vi "Periodic Tasks.vi"(8 "error in":errorcluster) -> ()   [LabVIEW 2019]
doc: "This VI runs in parallel to other tasks. It can contain as many user-defined periodic loops as you need. These can carry out PID or other sorts of timed response."
uses:
  <vilib>/Rock Robotics/WPI/ThirdParty/Phoenix-LabVIEW/Motor Controller/Get/CTRE_Phoenix_MotorController_GetSelectedSensorData.vi
  <vilib>/Rock Robotics/Network Tables/NT Write Number.vi
  <vilib>/Rock Robotics/WPI/ThirdParty/Phoenix-LabVIEW/Motor Controller/Get/CTRE_Phoenix_MotorController_GetQuadratureData.vi
  <vilib>/Rock Robotics/Network Tables/NT Read Number.vi
  <vilib>/Rock Robotics/Network Tables/NT Read Boolean.vi
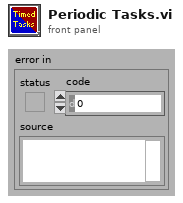
[diagram p1: front panel]
types:
  T1 = typedef "WPI_MotorControlDeviceRef.ctl" = cluster{"DeviceStatus":errorcluster, "Type":T2, "PWM":cluster{"PWM Channel":T3, "DeadBand":T4}, "CAN":cluster{"Device Number":u8, "SetOutput VI Ref":variant, "GetOutput VI Ref":variant, "Enable VI Ref":variant, "Disable VI Ref":variant, "Data":variant}, "Invert":bool, "DIO PWM":cluster{"PWM \"Enable\" Channel":T3, "DIOChannel":T5, "PWM Rate":dbl}}
  T2 = typedef "WPI_MotorControlType.ctl" = enum16{"PWM", "CAN", "DIO PWM"}
  T3 = typedef "FPGA_DIOPWMChannel.ctl" = enum8{"PWM 0", "PWM 1", "PWM 2", "PWM 3", "PWM 4", "PWM 5", "PWM 6", "PWM 7", "PWM 8", "PWM 9", "PWM MXP 0", "PWM MXP 1", "PWM MXP 2", "PWM MXP 3", "PWM MXP 4", "PWM MXP 5", "PWM MXP 6", "PWM MXP 7", "PWM MXP 8", "PWM MXP 9", "Invalid"}
  T4 = typedef "WPI_PWMDeadband.ctl" = cluster{"Name":string, "maxPositivePwm":i32, "minPositivePwm":i32, "centerPwm":i32, "maxNegativePwm":i32, "minNegativePwm":i32, "angularRange":u16}
  T5 = typedef "FPGA_DIOChannel.ctl" = enum8{"DIO 0", "DIO 1", "DIO 2", "DIO 3", "DIO 4", "DIO 5", "DIO 6", "DIO 7", "DIO 8", "DIO 9", "DIO MXP 0", "DIO MXP 1", "DIO MXP 2", "DIO MXP 3", "DIO MXP 4", "DIO MXP 5", "DIO MXP 6", "DIO MXP 7", "DIO MXP 8", "DIO MXP 9", "DIO MXP 10", "DIO MXP 11", "DIO MXP 12", "DIO MXP 13", "DIO MXP 14", "DIO MXP 15", "SPI Port CS1", "SPI Port CS2", "SPI Port CS3", "SPI Port MISO", "SPI Port MOSI", "Invalid"}
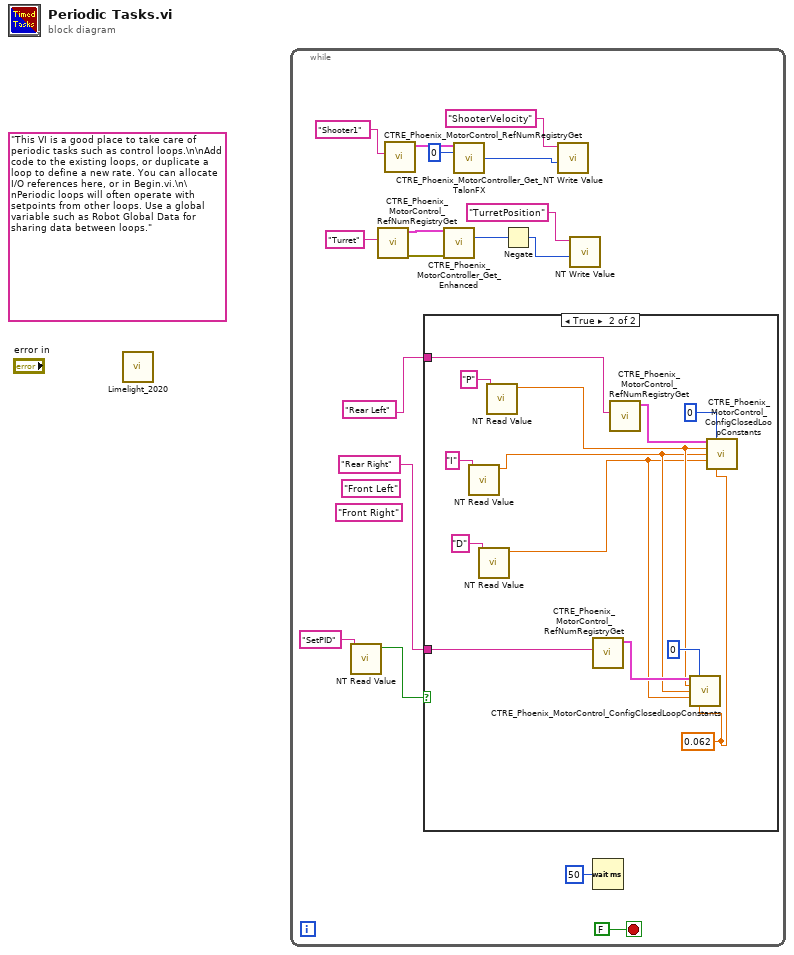
[diagram p0: block diagram]
diagram:
  (unwired) "This VI is a good place to take care of periodic tasks such as control loops.\n\nAdd code to the existing loops, or duplicate a loop to define a new rate. You can allocate I/O references here, or in Begin.vi.\n\nPeriodic loops will often operate with setpoints from other loops. Use a global variable such as Robot Global Data for sharing data between loops."
  n1 = call "Limelight_2020.vi"() -> ()  [unwired: 12 in]
  n2 = while {
    stop <- FALSE stop-if-true
    (unwired) "Front Right" ("refnum name")
    (unwired) "Front Left" ("refnum name")
    n3 = call-poly <vilib>:"NT Read Value.vi"("Name"="SetPID") -> ("Boolean"=w3:bool)  [unwired: 9 in, 1 out]
    n4 = call <vilib>:"CTRE_Phoenix_MotorControl_RefNumRegistryGet.vi"("refnum name"="Turret") -> ("error out"=w8:errorcluster, "PhoenixMotorControlDevRef"=w9:T1)  [unwired: 9 in]
    n5 = call <vilib>:"CTRE_Phoenix_MotorControl_RefNumRegistryGet.vi"("refnum name"="Shooter1") -> ("PhoenixMotorControlDevRef"=w15:T1)  [unwired: 9 in, 1 out]
    n6 = case shown="True" w3 {
      tunnel: "Rear Right" ("refnum name") -> [_ w25]
      tunnel: "Rear Left" ("refnum name") -> [_ w22]
      frame False {
      }
      frame True {
        w18 = 0.062 ("F")
        n7 = call-poly <vilib>:"NT Read Value.vi"("Name"="I") -> ("Numeric"=w20:dbl)  [unwired: 9 in, 1 out]
        n8 = call-poly <vilib>:"NT Read Value.vi"("Name"="D") -> ("Numeric"=w19:dbl)  [unwired: 9 in, 1 out]
        n9 = call-poly <vilib>:"NT Read Value.vi"("Name"="P") -> ("Numeric"=w21:dbl)  [unwired: 9 in, 1 out]
        n10 = call <vilib>:"CTRE_Phoenix_MotorControl_RefNumRegistryGet.vi"("refnum name"=w25) -> ("PhoenixMotorControlDevRef"=w24:T1)  [unwired: 9 in, 1 out]
        n11 = call <vilib>:"CTRE_Phoenix_MotorControl_RefNumRegistryGet.vi"("refnum name"=w22) -> ("PhoenixMotorControlDevRef"=w23:T1)  [unwired: 9 in, 1 out]
        n12 = call <vilib>:"CTRE_Phoenix_MotorControl_ConfigClosedLoopConstants.vi"("PhoenixMotorControlDevRef"=w24, "slotIdx"=0, "P"=w21, "I"=w20, "D"=w19, "F"=w18) -> ()  [unwired: 8 in, 2 out]
        n13 = call <vilib>:"CTRE_Phoenix_MotorControl_ConfigClosedLoopConstants.vi"("PhoenixMotorControlDevRef"=w23, "slotIdx"=0, "P"=w21, "I"=w20, "D"=w19, "F"=w18) -> ()  [unwired: 8 in, 2 out]
      }
    }
    n14 = call-poly <vilib>:"CTRE_Phoenix_MotorController_Get_Enhanced.vi"("PhoenixMotorControlDevRef"=w9, "error in"=w8) -> ("Quadrature Position"=w7:i32)  [unwired: 10 in, 3 out]
    n15 = call-poly <vilib>:"CTRE_Phoenix_MotorController_Get_TalonFX.vi"("PhoenixMotorControlDevRef"=w15, "pidLoopIdx"=u32 0) -> ("Velocity (Raw Sensor Units per 100 ms)"=w13:i32)  [unwired: 10 in, 3 out]
    n16 = Negate(x=w7) -> (-x=w5:i32)
    n17 = call-poly <vilib>:"NT Write Value.vi"("Numeric"=w13, "Name"="ShooterVelocity") -> ()  [unwired: 9 in, 1 out]
    n18 = call-poly <vilib>:"NT Write Value.vi"("Numeric"=w5, "Name"="TurretPosition") -> ()  [unwired: 9 in, 1 out]
    n19 = Wait (ms)(milliseconds to wait=u32 50) -> ()  [unwired: 1 out]
  }
